vi "Analyze Frequency Response of Filter.vi"() -> ()   [LabVIEW 2023]
doc: "Demonstrates how to use the Filter Analysis VIs to analyze the frequency response of the designed filter.\n\nComplete the following steps to use this VI.\n1) Run the VI.\n2) Observe the plots on the Magnitude Response, Phase Response, and Group Delay graphs.\n3) Change the specifications and observe the characteristics of the filter you just designed.\n4) Click the <B>STOP</B> button to stop this VI."
uses:
  <vilib>/addons/Digital Filter Design/_Objects.llb/DFD Filter Ripple Specification (Design).ctl
  <vilib>/addons/Digital Filter Design/_Objects.llb/DFD Filter Frequence Specification (Design).ctl
  <vilib>/addons/Digital Filter Design/_Objects.llb/DFD Phase Setting.ctl
  <vilib>/addons/Digital Filter Design/Analysis.llb/DFD Plot Freq Response (Linear-Spaced).vi
  <vilib>/addons/Digital Filter Design/NI_DigFilterLicensed.lvlib
panel:
  in  "Design Method":T1(ring)=enum."Elliptic"
  in  "Analysis Tab":T2(tab)
  in  "dB on?":bool=TRUE
  out "Magnitude Response":cluster{"f0":dbl, "df":dbl, "values":dbl[]}[](graph)
  in  "phase view":T3={"unwrap? (F)"=TRUE, "degree? (F)"=FALSE}
  out "Phase Response":cluster{"f0":dbl, "df":dbl, "values":dbl[]}[](graph)
  out "Group Delay":cluster{"f0":dbl, "df":dbl, "values":dbl[]}[](graph)
  in  "Filter Type":u16(ring) items=["Lowpass", "Highpass", "Bandpass", "Bandstop"]
  in  "Frequency Sepcifications [Hz]":T4={"fpass 1"=100.0, "fstop 1"=200.0, "fpass 2 "=0.0, "fstop 2"=0.0}
  in  "Ripple Specifications":T5={"passband"=0.1, "stopband"=60.0, "dB/linear? (T: dB)"=TRUE}
  in  "Sampling Frequency [Hz]":dbl=1000.0 format="%.2f"
  in  "stop":bool
  out "Error Message":string
  # "Select Help>>Show Context Help and move the cursor over the VI icon for more information."
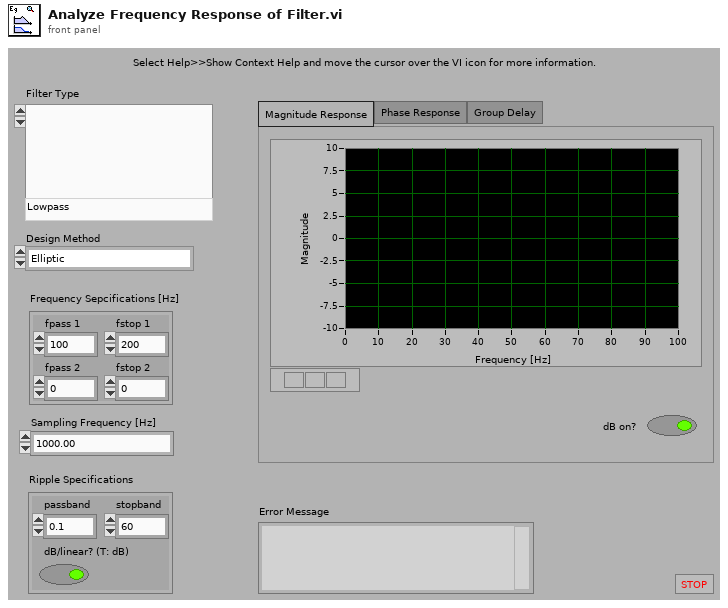
[diagram p1: front panel]
types:
  T1 = enum16{"Butterworth", "Chebyshev", "Inverse Chebyshev", "Elliptic", "Kaiser Window", "Dolph-Chebyshev Window", "Equi-Ripple FIR"}
  T2 = enum32{"Magnitude Response", "Phase Response", "Group Delay"}
  T3 = typedef "NI_DigFilterLicensed.lvlib/DFD Phase Setting.ctl" = cluster{"unwrap? (F)":bool, "degree? (F)":bool}
  T4 = typedef "NI_DigFilterLicensed.lvlib/DFD Filter Frequence Specification (Design).ctl" = cluster{"fpass 1":dbl, "fstop 1":dbl, "fpass 2 ":dbl, "fstop 2":dbl}
  T5 = typedef "NI_DigFilterLicensed.lvlib/DFD Filter Ripple Specification (Design).ctl" = cluster{"passband":dbl, "stopband":dbl, "dB/linear? (T: dB)":bool}
  T6 = typedef "NI_DigFilterLicensed.lvlib/DFD Filter Obj.ctl" = cluster{"mSRate_Fs":dbl, "mSRate_Version":string, "mSRate_Comments":string, "mSRate_OrgCoef":T7, "mSRate_CurCoef":T7, "mSRate_Quantized?":bool, "mSRate_QCoef":T7, "mSRate_QSettings":T9[], "mSRate_Order":i32, "mSRate_Scaling":cluster{"mSRate_ScaleByPowerOf2?":bool, "mSRate_ScaleType":T11}}
  T7 = typedef "NI_DigFilterLicensed.lvlib/DFD Filter Coef.ctl" = cluster{"type":T8, "gain":dbl, "coef a (k)":dbl[], "coef b (v)":dbl[]}
  T8 = typedef "NI_DigFilterLicensed.lvlib/DFD Filter Structure Type Selector.ctl" = enum16{"Undefined", "FIR Direct Form", "FIR Direct Form Transposed", "FIR Symmetric", "FIR Antisymmetric", "IIR Direct Form I", "IIR Direct Form I Transposed", "IIR Direct Form II", "IIR Direct Form II Transposed", "IIR Cascaded Second Order Sections Form I", "IIR Cascaded Second Order Sections Form I Transposed", "IIR Cascaded Second Order Sections Form II", "IIR Cascaded Second Order Sections Form II Transposed", "Lattice Allpass (basic sections)", "Lattice Allpass (one multiplier sections)", "Lattice Allpass (normalized sections)", "Lattice AR (basic sections)", "Lattice AR (one multiplier sections)", "Lattice AR (normalized sections)", "Lattice MA (minimum phase)", "Lattice MA (maximum phase)", "Lattice ARMA (basic sections)", "Lattice ARMA (one multiplier sections)", "Lattice ARMA (normalized sections)"}
  T9 = typedef "NI_DigFilterLicensed.lvlib/dfd_Internal Quantization Settings.ctl" = cluster{"source":T10, "wl":i16, "iwl":i16, "overflow mode":enum16{"Saturation", "Wrap"}, "rounding mode":enum16{"Nearest", "Truncation"}, "signed?":bool}
  T10 = typedef "NI_DigFilterLicensed.lvlib/dfd_Internal Quantization Srcs.ctl" = u16
  T11 = typedef "NI_DigFilterLicensed.lvlib/DFD Coef Norm Type.ctl" = enum16{"No Norm", "Time Domain 1-Norm", "Time Domain 2-Norm", "Time Domain Inf-Norm"}
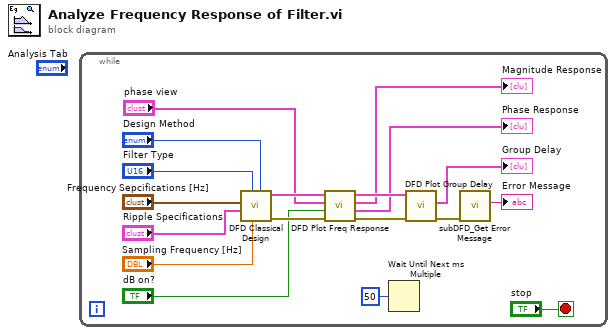
[diagram p0: block diagram]
diagram:
  n1 = while {
    stop <- "stop" stop-if-true
    n2 = call <vilib>:"DFD Classical Design.vi"("design method"="Design Method", "fs [Hz]"="Sampling Frequency [Hz]", "filter type"="Filter Type", "ripple specs"="Ripple Specifications", "freq specs [Hz]"="Frequency Sepcifications [Hz]") -> ("error out"=w12:errorcluster, "filter out"=w13:T6)  [unwired: 1 in, 4 out]
    n3 = call-poly <vilib>:"DFD Plot Freq Response.vi"("error in (no error)"=w12, "dB on? (T)"="dB on?", "phase view"="phase view", "filter in"=w13) -> ("error out"=w10:errorcluster, "phase response"=→"Phase Response":cluster{"f0":dbl, "df":dbl, "values":dbl[]}[], "magnitude response"=→"Magnitude Response":cluster{"f0":dbl, "df":dbl, "values":dbl[]}[], "filter out"=w11:T6)  [unwired: 4 in]
    n4 = Wait Until Next ms Multiple(millisecond multiple=u32 50) -> ()  [unwired: 1 out]
    n5 = call <vilib>:"DFD Plot Group Delay.vi"("error in (no error)"=w10, "filter in"=w11) -> ("error out"=w3:errorcluster, "group delay"=→"Group Delay":cluster{"f0":dbl, "df":dbl, "values":dbl[]}[])  [unwired: 2 in, 6 out]
    n6 = call <vilib>:"subDFD_Get Error Message.vi"("error in (no error)"=w3) -> ("Error Message"=→"Error Message":string)  [unwired: 1 in, 9 out]
  }
